vi "H5Gget_objname_by_idx.vi"(6 "error in (no error)":errorcluster, 8 "Index":u64, 9 "HDF5 Ref":T1) -> (0 "error out":errorcluster, 2 "Name":string, 3 "HDF5 Ref out":T1)   [LabVIEW 2017]
doc: "Returns a name of an object specified by an index."
uses:
  <vilib>/UPVI/lvhdf5/library.llb/HDF5 Ref.ctl
  <vilib>/UPVI/lvhdf5/hdf5.dll
panel:
  # "LVHDF5 Toolkit\nCopyright (c) 2005-2013 by Jason D. Sommerville\nCopyright (c) 2014 by UPVI, LLC.\n\nThis use and distribution of this file is governed by the terms found in \nLICENSE.txt distributed with this toolkit and installed at\n <user.lib>\\_lvhdf5\\LICENSE.txt"
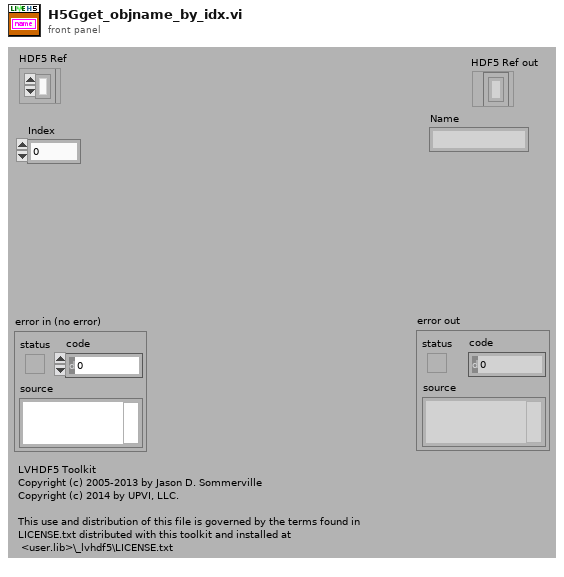
[diagram p1: front panel]
types:
  T1 = typedef "HDF5 Ref.ctl" = refnum<k1>
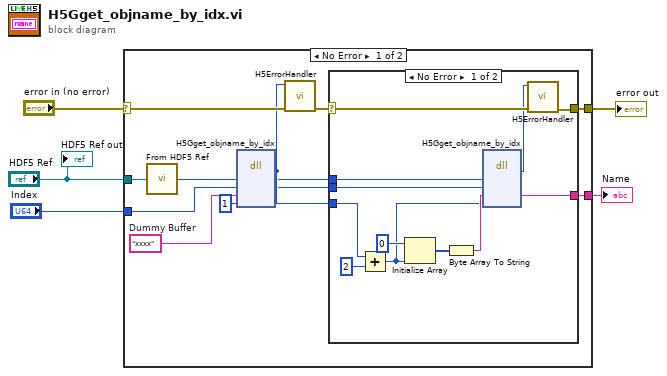
[diagram p0: block diagram]
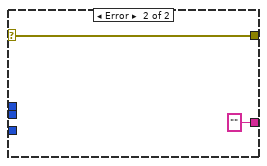
[diagram p2: hidden frame]
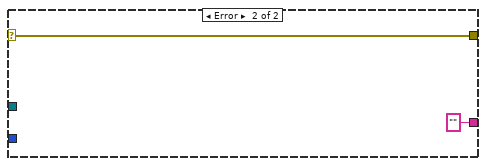
[diagram p3: hidden frame]
diagram:
  n1 = case shown="No Error" "error in (no error)" {
    selector: "error in (no error)" -> [w17 w33]
    tunnel: [w11 w33] -> w4
    tunnel: "HDF5 Ref" -> [w16 _]
    tunnel: "Index" -> [w6 _]
    tunnel: [w7 "" ("name")] -> w1
    frame No Error {
      w14 = "xxxx"  # Dummy Buffer
      n2 = call <vilib>:"From HDF5 Ref.vi"("HDF5 Ref"=w16) -> ("I32"=w15:i32)
      n3 = dll-call lib="C:/Program Files/National Instruments/LabVIEW 2017/vi.lib/UPVI/lvhdf5/hdf5.dll" fn="H5Gget_objname_by_idx"("loc_id"=w15, "idx"=w6, "name"=w14, "size"=u32 1) -> ("return type"=w10:i64, "loc_id"=w8:i32, "idx"=w9:u64)  [unwired: 5 in, 2 out]
      n4 = call <vilib>:"H5ErrorHandler.vi"("error in (no error)"=w17, "herr_t"=w10) -> ("error out"=w12:errorcluster)  [unwired: 3 in, 4 out]
      n5 = case shown="No Error" w12 {
        selector: w12 -> [w22 w31]
        tunnel: [w23 w31] -> w11
        tunnel: w10 -> [w19 _]
        tunnel: w9 -> [w25 _]
        tunnel: w8 -> [w24 _]
        tunnel: [w20 "" ("name")] -> w7
        frame No Error {
          n6 = Add(x=w19, y=2) -> (x+y=w18:i64)
          n7 = Initialize Array(u8 0, w18) -> (w27:u8[])
          n8 = Byte Array To String(unsigned byte array=w27) -> (string=w26:string)
          n9 = dll-call lib="C:/Program Files/National Instruments/LabVIEW 2017/vi.lib/UPVI/lvhdf5/hdf5.dll" fn="H5Gget_objname_by_idx"("loc_id"=w24, "idx"=w25, "name"=w26, "size"=w18) -> ("return type"=w21:i64, "name"=w20:string)  [unwired: 6 in, 2 out]
          n10 = call <vilib>:"H5ErrorHandler.vi"("error in (no error)"=w22, "herr_t"=w21) -> ("error out"=w23:errorcluster)  [unwired: 3 in, 4 out]
        }
        frame Error {
        }
      }
    }
    frame Error {
    }
  }
  "error out" <- w4
  "Name" <- w1
  "HDF5 Ref out" <- "HDF5 Ref"
